vi "ExamplePlugin.vi"() -> ()   [LabVIEW 2024, in "ExamplePlugin.lvlib"]
uses:
  ExamplePlugin.lvlib
  Plugin SDK/Plugin Events Enum.ctl
  Plugin SDK/Write Edit Time Configuration.vi
  Plugin SDK/Write Run Time Configuration.vi
  Plugin SDK/Read Edit Time Configuration.vi
  Plugin SDK/Read Run Time Configuration.vi
  Plugin SDK/Plugin Session.lvclass
  Plugin SDK/InstrumentStudio Plugin SDK.lvlib
panel:
  in  "Tab Control 2":T1(tab)
  in  "Read Selected Sites":bool
  in  "Read Active Pin Map Path":bool
  out "Sites":i32[](array[numeric])
  out "Project Path":path
  in  "Run Write":string
  in  "Write Run Time Config":bool
  in  "Edit Write":string
  in  "Write Edit Time Config":bool
  out "Run Read":string
  in  "Read Run Time Config":bool
  out "Edit Read":string
  in  "Read Edit Time Config":bool
  in  "Read Project Path":bool
  in  "Running":bool
  out "Active Pin Map Path":path
  out "Event Record":i32(listbox)
  in  "Session Id":u64
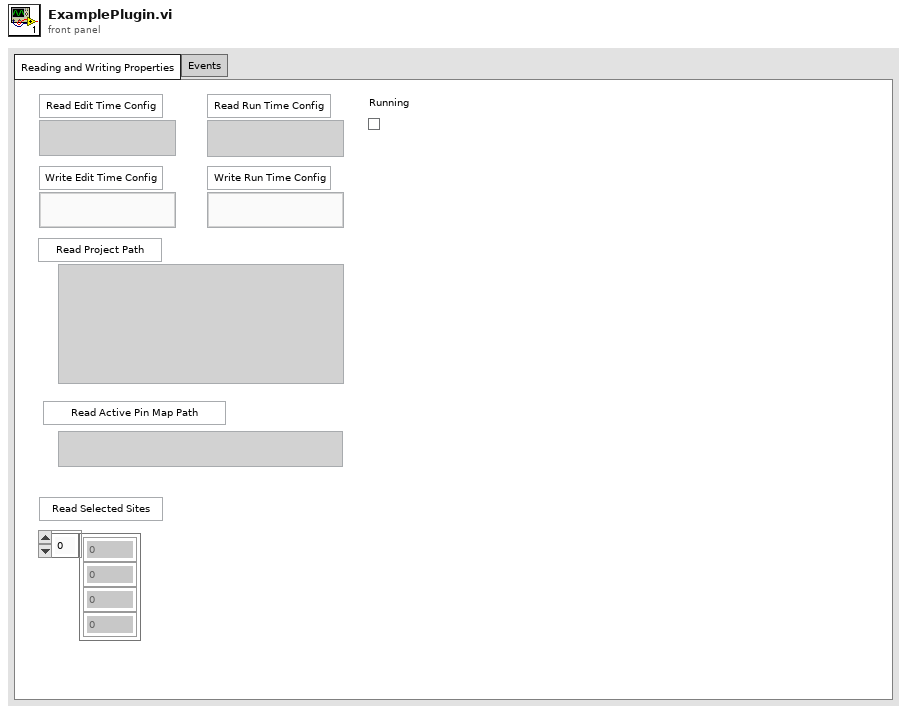
[diagram p1: front panel]
types:
  T1 = enum32{"Reading and Writing Properties", "Events"}
  T2 = typedef "InstrumentStudio Plugin SDK.lvlib/Plugin Events Enum.ctl" = enum32{"Shutdown", "Project Saved", "Stop All Outputs", "Generic Message", "Active Pin Map Changed", "Selected Sites Changed"}
  T3 = typedef "InstrumentStudio Plugin SDK.lvlib/Event Registration Refnum.ctl" = refnum<event-registration>
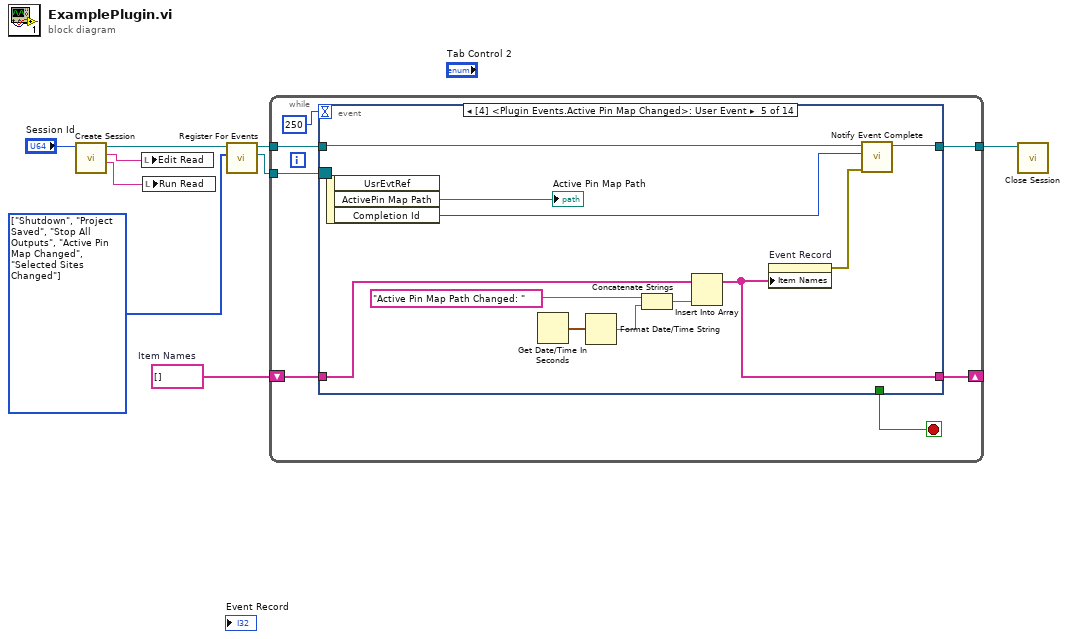
[diagram p0: block diagram]
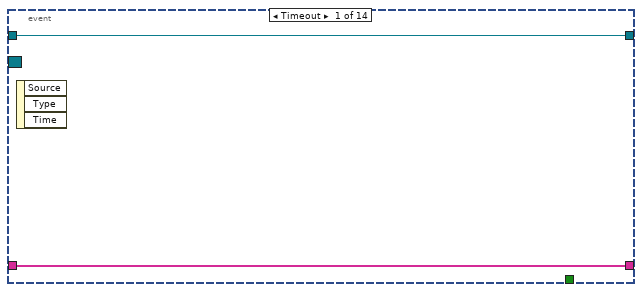
[diagram p2: hidden frame]
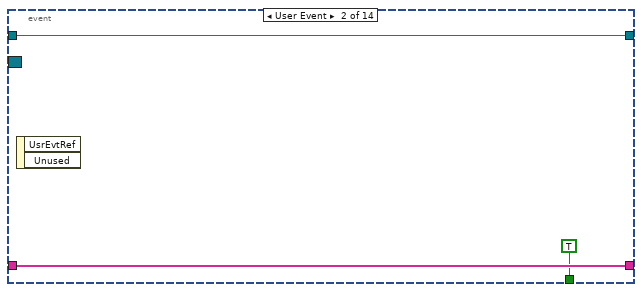
[diagram p3: hidden frame]
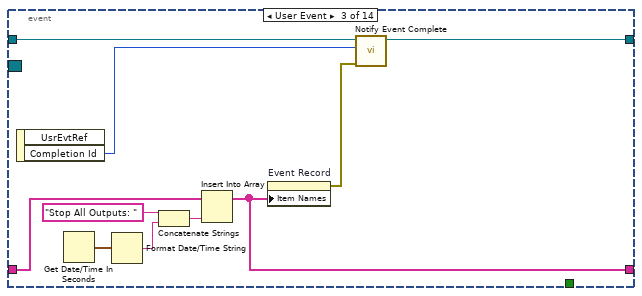
[diagram p4: hidden frame]
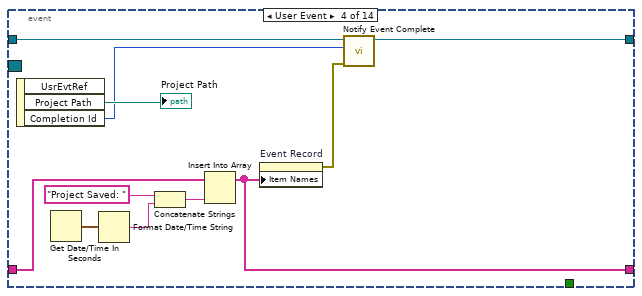
[diagram p5: hidden frame]
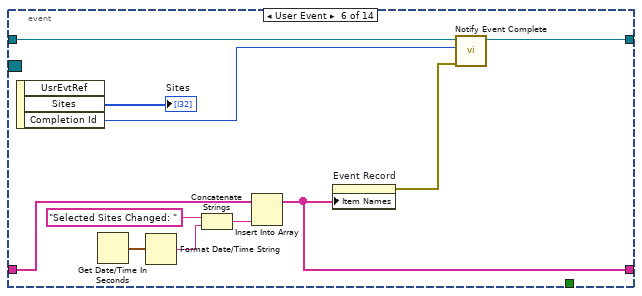
[diagram p6: hidden frame]
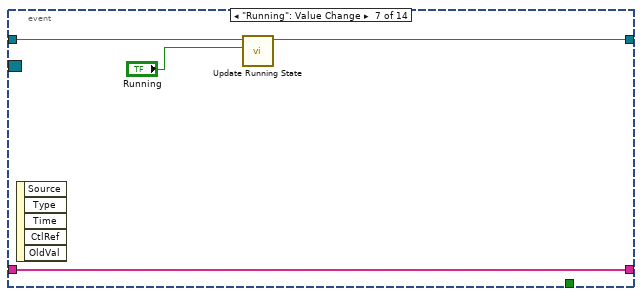
[diagram p7: hidden frame]
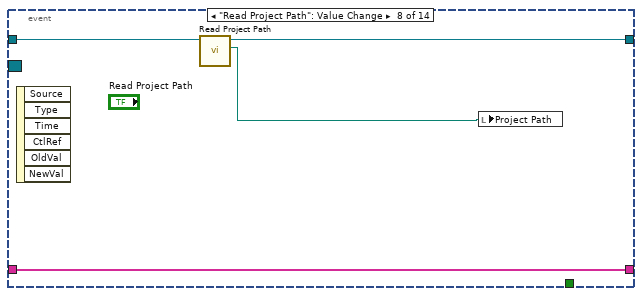
[diagram p8: hidden frame]
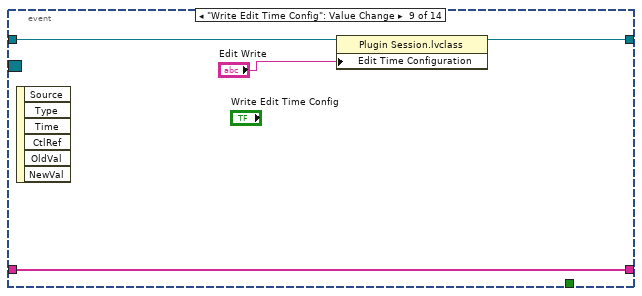
[diagram p9: hidden frame]
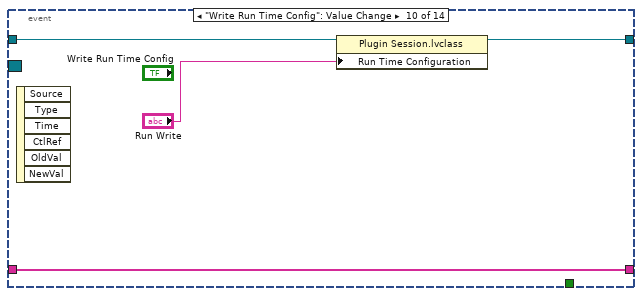
[diagram p10: hidden frame]
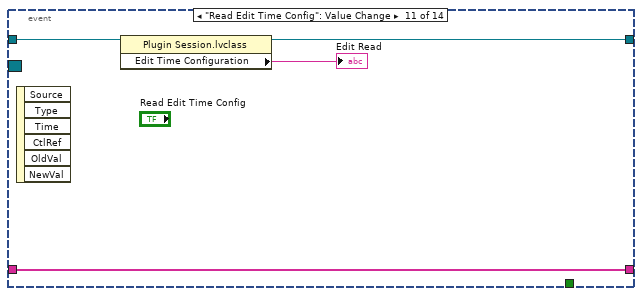
[diagram p11: hidden frame]
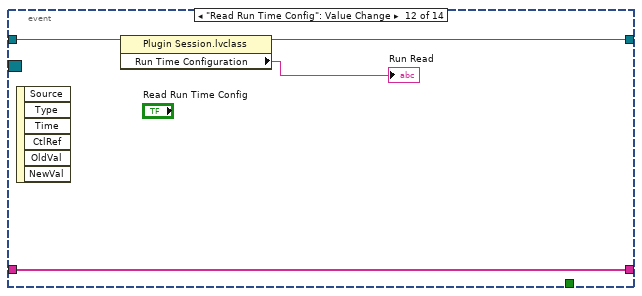
[diagram p12: hidden frame]
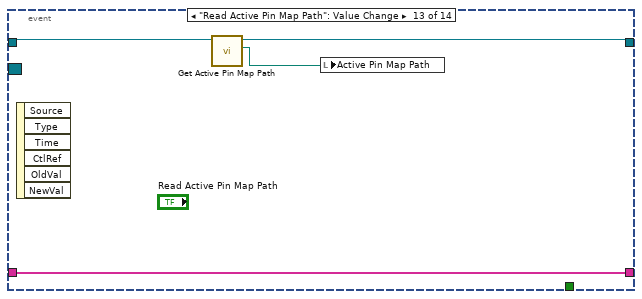
[diagram p13: hidden frame]
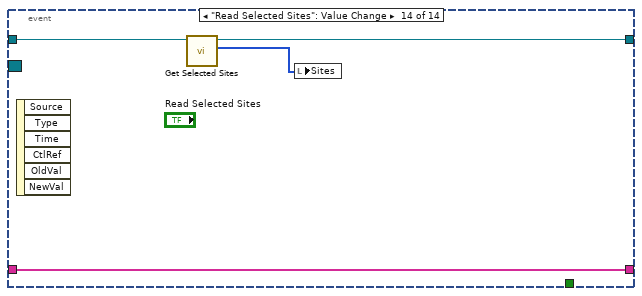
[diagram p14: hidden frame]
diagram:
  w4 = T2[] [enum."Shutdown", enum."Project Saved", enum."Stop All Outputs", enum."Active Pin Map Changed", enum."Selected Sites Changed"] items=["Shutdown", "Project Saved", "Stop All Outputs", "Generic Message", "Active Pin Map Changed", "Selected Sites Changed"] ("Events To Register")
  w7 = string[] []  # Item Names
  n1 = call "Create Session.vi"("Session Id"="Session Id") -> ("Run Time Configuration"=w2:string, "Edit Time Configuration"=w1:string, "Session out"=w8:refnum<class "Plugin Session.lvclass">)  [unwired: 6 in, 2 out]
  n2 = local write "Edit Read"(w1) -> ()
  n3 = local write "Run Read"(w2) -> ()
  n4 = call "Register For Events.vi"("Events To Register"=w4, "Session in"=w8) -> ("Event Refnum"=w3:T3, "Session out"=w6:refnum<class "Plugin Session.lvclass">)  [unwired: 7 in, 1 out]
  n5 = while {
    shift-right: [w14] -> _
    shift-left: w7 -> [w15]
    tunnel: w6 -> [w13]
    tunnel: [w12] -> w5
    tunnel: w3 -> [w11]
    stop <- w10 stop-if-true
    n6 = event shown="[4] <Plugin Events.Active Pin Map Changed>: User Event" {
      selector: w11 -> [_ _ _ _ _ _ _ _ _ _ _ _ _ _]
      dyn-events: _ -> [_ _ _ _ _ _ _ _ _ _ _ _ _ _]
      timeout: 250 -> [_ _ _ _ _ _ _ _ _ _ _ _ _ _]
      tunnel: w15 -> [w18 w21 w27 w40 w48 w60 w68 w72 w76 w80 w84 w88 w92 w96]
      tunnel: [w18 w21 w26 w36 w47 w59 w68 w72 w76 w80 w84 w88 w92 w96] -> w14
      tunnel: w13 -> [w17 w19 w25 w34 w45 w57 w67 w71 w75 w79 w83 w87 w89 w95]
      tunnel: [w17 w19 w24 w33 w44 w58 w66 w70 w73 w77 w81 w85 w90 w94] -> w12
      tunnel: [_ TRUE _ _ _ _ _ _ _ _ _ _ _ _] -> w10
      event Timeout {
        n7 = event-data() -> ()  [unwired: 1 in, 3 out]
      }
      event User Event {
        n8 = event-data() -> ()  [unwired: 1 in, 2 out]
      }
      event User Event {
        n9 = event-data() -> ("Completion Id"=w23:i64)  [unwired: 1 in, 1 out]
        n10 = Get Date/Time In Seconds() -> (seconds since 1Jan1904=w28:timestamp)
        n11 = Format Date/Time String(seconds (now)=w28) -> (date/time string=w30:string)  [unwired: 2 in]
        n12 = Concatenate Strings("Stop All Outputs: ", w30) -> (w29:string)
        n13 = Insert Into Array(array=w27, new element=w29) -> (w26:string[])  [unwired: 1 in]
        n14 = property on="Event Record" class="LstBox (strict)"("Item Names"=w26) -> (error out=w22:errorcluster)  [unwired: 2 in, 1 out]
        n15 = call "Notify Event Complete.vi"("error in (no error)"=w22, "Completion Id"=w23, "Session in"=w25) -> ("Session out"=w24:refnum<class "Plugin Session.lvclass">)  [unwired: 7 in, 1 out]
      }
      event User Event {
        n16 = event-data() -> ("Project Path"=→"Project Path":path, "Completion Id"=w41:i64)  [unwired: 1 in, 1 out]
        n17 = Get Date/Time In Seconds() -> (seconds since 1Jan1904=w35:timestamp)
        n18 = Format Date/Time String(seconds (now)=w35) -> (date/time string=w38:string)  [unwired: 2 in]
        n19 = Concatenate Strings("Project Saved: ", w38) -> (w37:string)
        n20 = Insert Into Array(array=w40, new element=w37) -> (w36:string[])  [unwired: 1 in]
        n21 = property on="Event Record" class="LstBox (strict)"("Item Names"=w36) -> (error out=w32:errorcluster)  [unwired: 2 in, 1 out]
        n22 = call "Notify Event Complete.vi"("error in (no error)"=w32, "Completion Id"=w41, "Session in"=w34) -> ("Session out"=w33:refnum<class "Plugin Session.lvclass">)  [unwired: 7 in, 1 out]
      }
      event User Event {
        n23 = event-data() -> ("ActivePin Map Path"=→"Active Pin Map Path":path, "Completion Id"=w43:i64)  [unwired: 1 in, 1 out]
        n24 = Get Date/Time In Seconds() -> (seconds since 1Jan1904=w50:timestamp)
        n25 = Format Date/Time String(seconds (now)=w50) -> (date/time string=w52:string)  [unwired: 2 in]
        n26 = Concatenate Strings("Active Pin Map Path Changed: ", w52) -> (w51:string)
        n27 = Insert Into Array(array=w48, new element=w51) -> (w47:string[])  [unwired: 1 in]
        n28 = property on="Event Record" class="LstBox (strict)"("Item Names"=w47) -> (error out=w49:errorcluster)  [unwired: 2 in, 1 out]
        n29 = call "Notify Event Complete.vi"("error in (no error)"=w49, "Completion Id"=w43, "Session in"=w45) -> ("Session out"=w44:refnum<class "Plugin Session.lvclass">)  [unwired: 7 in, 1 out]
      }
      event User Event {
        n30 = event-data() -> ("Sites"=→"Sites":i32[], "Completion Id"=w54:i64)  [unwired: 1 in, 1 out]
        n31 = Get Date/Time In Seconds() -> (seconds since 1Jan1904=w61:timestamp)
        n32 = Format Date/Time String(seconds (now)=w61) -> (date/time string=w63:string)  [unwired: 2 in]
        n33 = Concatenate Strings("Selected Sites Changed: ", w63) -> (w62:string)
        n34 = Insert Into Array(array=w60, new element=w62) -> (w59:string[])  [unwired: 1 in]
        n35 = property on="Event Record" class="LstBox (strict)"("Item Names"=w59) -> (error out=w55:errorcluster)  [unwired: 2 in, 1 out]
        n36 = call "Notify Event Complete.vi"("error in (no error)"=w55, "Completion Id"=w54, "Session in"=w57) -> ("Session out"=w58:refnum<class "Plugin Session.lvclass">)  [unwired: 7 in, 1 out]
      }
      event "Running": Value Change {
        n37 = event-data() -> ()  [unwired: 1 in, 5 out]
        n38 = call "Update Running State.vi"("Is Running"="Running", "Plugin Session in"=w67) -> ("Plugin Session out"=w66:refnum<class "Plugin Session.lvclass">)  [unwired: 8 in, 1 out]
      }
      event "Read Project Path": Value Change {
        n39 = event-data() -> ()  [unwired: 1 in, 6 out]
        n40 = call "Read Project Path.vi"("Session in"=w71) -> ("Project Path"=w69:path, "Session out"=w70:refnum<class "Plugin Session.lvclass">)  [unwired: 8 in, 1 out]
        n41 = local write "Project Path"(w69) -> ()
      }
      event "Write Edit Time Config": Value Change {
        n42 = event-data() -> ()  [unwired: 1 in, 6 out]
        n43 = property class="Plugin Session.lvclass"(reference=w75, "Edit Time Configuration"="Edit Write") -> (reference out=w73:refnum<class "Plugin Session.lvclass">)  [unwired: 1 in, 1 out]
      }
      event "Write Run Time Config": Value Change {
        n44 = event-data() -> ()  [unwired: 1 in, 6 out]
        n45 = property class="Plugin Session.lvclass"(reference=w79, "Run Time Configuration"="Run Write") -> (reference out=w77:refnum<class "Plugin Session.lvclass">)  [unwired: 1 in, 1 out]
      }
      event "Read Edit Time Config": Value Change {
        n46 = event-data() -> ()  [unwired: 1 in, 6 out]
        n47 = property class="Plugin Session.lvclass"(reference=w83) -> (reference out=w81:refnum<class "Plugin Session.lvclass">, "Edit Time Configuration"=→"Edit Read":string)  [unwired: 1 in, 1 out]
      }
      event "Read Run Time Config": Value Change {
        n48 = event-data() -> ()  [unwired: 1 in, 6 out]
        n49 = property class="Plugin Session.lvclass"(reference=w87) -> (reference out=w85:refnum<class "Plugin Session.lvclass">, "Run Time Configuration"=→"Run Read":string)  [unwired: 1 in, 1 out]
      }
      event "Read Active Pin Map Path": Value Change {
        n50 = event-data() -> ()  [unwired: 1 in, 6 out]
        n51 = call-dynamic "Get Active Pin Map Path.vi"("Session in"=w89) -> ("Active Pin Map Path"=w91:path, "Session out"=w90:refnum<class "Plugin Session.lvclass">)  [unwired: 8 in, 1 out]
        n52 = local write "Active Pin Map Path"(w91) -> ()
      }
      event "Read Selected Sites": Value Change {
        n53 = event-data() -> ()  [unwired: 1 in, 6 out]
        n54 = call-dynamic "Get Selected Sites.vi"("Session in"=w95) -> ("Selected Sites"=w93:i32[], "Session out"=w94:refnum<class "Plugin Session.lvclass">)  [unwired: 8 in, 1 out]
        n55 = local write "Sites"(w93) -> ()
      }
    }
  }
  n56 = call "Close Session.vi"("Session in"=w5) -> ()  [unwired: 10 in, 1 out]
